vi "read_config_file.vi"(8 "error in (no error)":errorcluster, 11 "Application Directory":path) -> (0 "error out":errorcluster, 1 "gui_strings":string[](array[string]), 2 "devices":T1, 3 "gral_config":T3={"file_ext"="0.0.0.0", "TCP port"=0, "#devices"=0, "log?"=FALSE, "tcp?"=FALSE, "language"="ENG"})   [LabVIEW 2013]
doc: "Reads the configuration file (config.ini)"
uses:
  type_def/general.ctl
  type_def/device_array.ctl
  type_def/device.ctl
  <vilib>/Utility/config.llb/Read Key (I32).vi
  <vilib>/Utility/config.llb/Read Key (Boolean).vi
  <vilib>/Utility/config.llb/Read Key (String).vi
  <vilib>/Utility/config.llb/Read Key (Path).vi
  <vilib>/Utility/config.llb/NI_LVConfig.lvlib
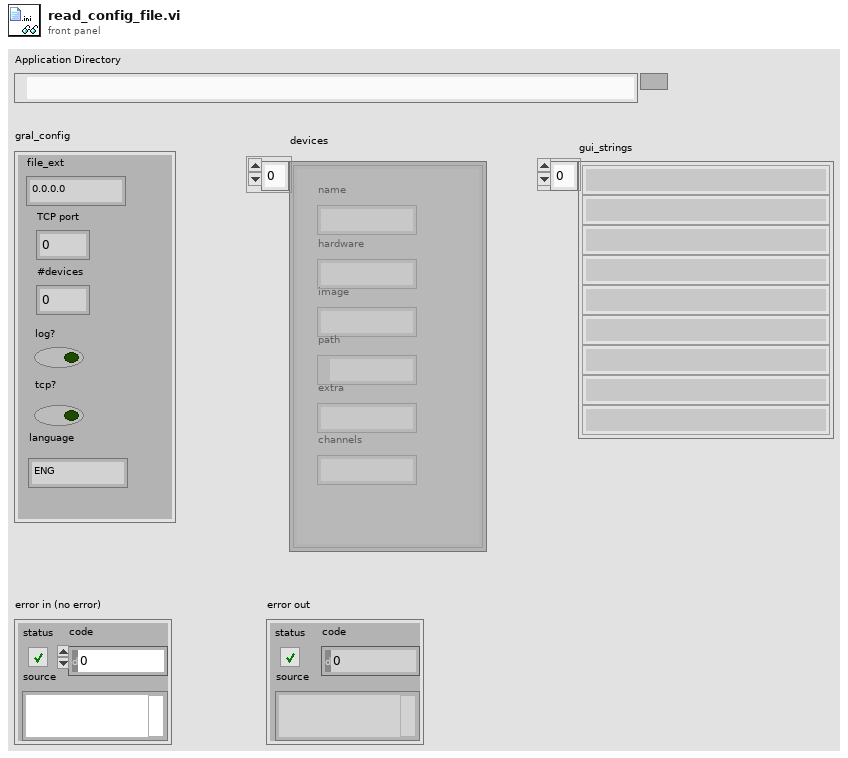
[diagram p1: front panel]
types:
  T1 = typedef "device_array.ctl" = T2[]
  T2 = typedef "device.ctl" = cluster{"name":string, "hardware":string, "image":string, "path":path, "extra":string, "channels":string}
  T3 = typedef "general.ctl" = cluster{"file_ext":string, "TCP port":i32, "#devices":i32, "log?":bool, "tcp?":bool, "language":string}
  T4 = typedef "NI_LVConfig.lvlib/Config Data RefNum.ctl" = refnum<k1>
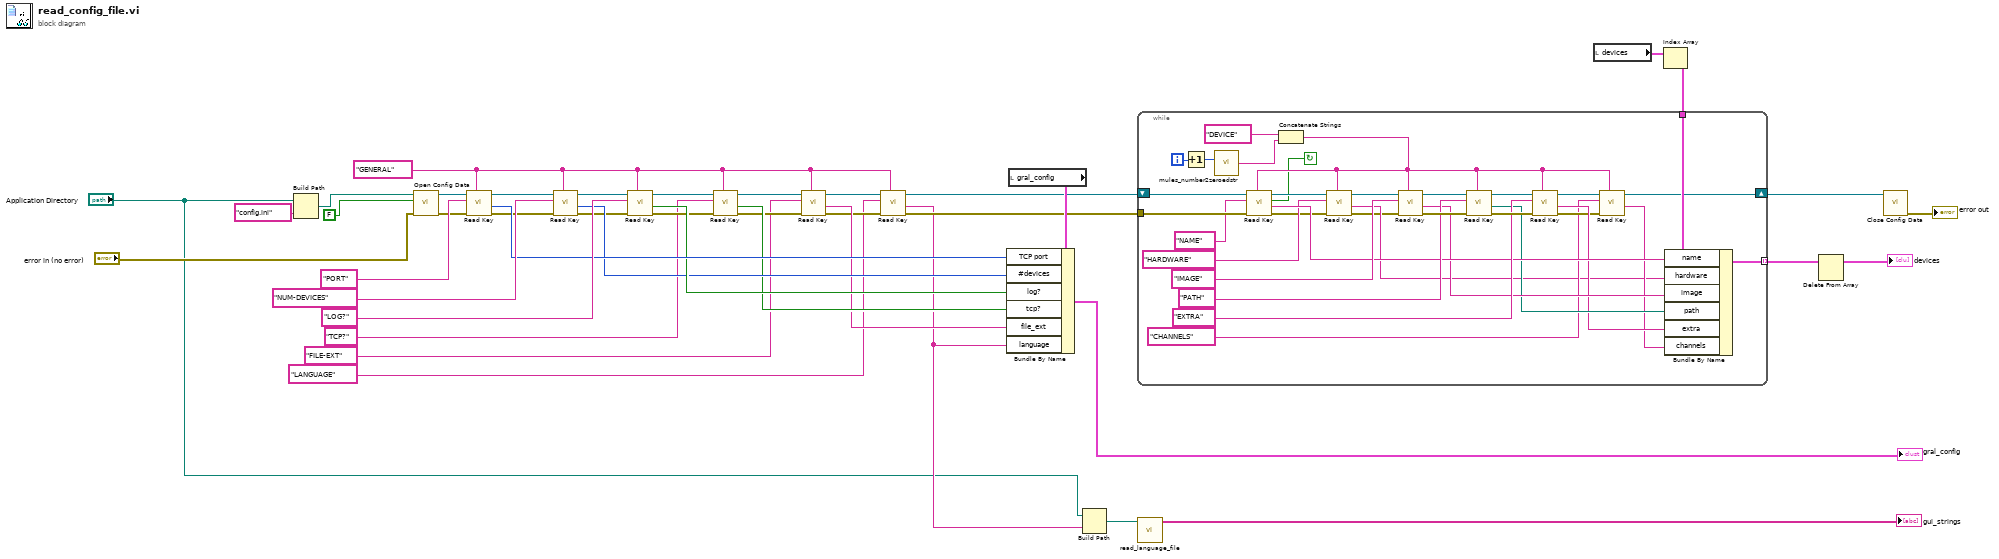
[diagram p0: block diagram]
diagram:
  w13 = "GENERAL" ("section")
  n1 = Build Path(base path="Application Directory", name or relative path="config.ini") -> (appended path=w41:path)
  n2 = call <vilib>:"Open Config Data.vi"("error in (no error)"="error in (no error)", "create file if necessary (T)"=FALSE, "configuration file path"=w41) -> ("error out"=w6:errorcluster, "refnum"=w9:T4)  [unwired: 6 in, 1 out]
  n3 = call-poly <vilib>:"Read Key.vi"("section"=w13, "error in (no error)"=w6, "key"="PORT", "refnum"=w9) -> ("error out"=w7:errorcluster, "value"=w33:i32, "refnum out"=w8:T4)  [unwired: 4 in, 1 out]
  n4 = call-poly <vilib>:"Read Key.vi"("section"=w13, "error in (no error)"=w7, "key"="NUM-DEVICES", "refnum"=w8) -> ("error out"=w27:errorcluster, "value"=w31:i32, "refnum out"=w37:T4)  [unwired: 4 in, 1 out]
  n5 = call-poly <vilib>:"Read Key.vi"("section"=w13, "error in (no error)"=w27, "key"="LOG?", "refnum"=w37) -> ("error out"=w24:errorcluster, "value"=w32:bool, "refnum out"=w25:T4)  [unwired: 4 in, 1 out]
  n6 = call-poly <vilib>:"Read Key.vi"("section"=w13, "error in (no error)"=w24, "key"="TCP?", "refnum"=w25) -> ("error out"=w20:errorcluster, "value"=w22:bool, "refnum out"=w21:T4)  [unwired: 4 in, 1 out]
  n7 = call-poly <vilib>:"Read Key.vi"("section"=w13, "error in (no error)"=w20, "key"="FILE-EXT", "refnum"=w21) -> ("error out"=w17:errorcluster, "value"=w18:string, "refnum out"=w14:T4)  [unwired: 4 in, 1 out]
  n8 = call-poly <vilib>:"Read Key.vi"("section"=w13, "error in (no error)"=w17, "key"="LANGUAGE", "refnum"=w14) -> ("error out"=w16:errorcluster, "value"=w4:string, "refnum out"=w15:T4)  [unwired: 4 in, 1 out]
  n9 = local read "gral_config"() -> (w34:T3)
  n10 = Bundle By Name(cluster=w34, "TCP port"=w33, "#devices"=w31, "log?"=w32, "tcp?"=w22, "file_ext"=w18, "language"=w4) -> (→"gral_config":T3)
  n11 = Build Path(base path="Application Directory", name or relative path=w4) -> (appended path=w5:path)
  n12 = call "read_language_file.vi"("Text File"=w5) -> ("gui_strings"=→"gui_strings":string[])  [unwired: 10 in]
  n13 = local read "devices"() -> (w30:T1)
  n14 = Index Array(array=w30) -> (element=w29:T2)  [unwired: 1 in]
  n15 = while {
    shift-right: [w54] -> w38
    shift-left: w15 -> [w73]
    tunnel: w29 -> [w61]
    tunnel: [w60] -> w11 mode=indexing
    tunnel: w16 -> [w68]
    i -> [w75]
    stop <- w43 continue-if-true
    n16 = Increment(x=w75) -> (x+1=w74:i32)
    n17 = call "mules_number2zeroedstr.vi"("number"=w74) -> ("string"=w62:string)  [unwired: 1 in]
    n18 = Concatenate Strings("DEVICE" ("key"), w62) -> (w48:string)
    n19 = call-poly <vilib>:"Read Key.vi"("section"=w48, "error in (no error)"=w68, "key"="NAME", "refnum"=w73) -> ("error out"=w45:errorcluster, "value"=w59:string, "found?"=w43:bool, "refnum out"=w50:T4)  [unwired: 4 in]
    n20 = call-poly <vilib>:"Read Key.vi"("section"=w48, "error in (no error)"=w45, "key"="HARDWARE", "refnum"=w50) -> ("error out"=w44:errorcluster, "value"=w46:string, "refnum out"=w49:T4)  [unwired: 4 in, 1 out]
    n21 = call-poly <vilib>:"Read Key.vi"("section"=w48, "error in (no error)"=w44, "key"="IMAGE", "refnum"=w49) -> ("error out"=w69:errorcluster, "value"=w58:string, "refnum out"=w72:T4)  [unwired: 4 in, 1 out]
    n22 = call-poly <vilib>:"Read Key.vi"("section"=w48, "error in (no error)"=w69, "key"="PATH", "refnum"=w72) -> ("error out"=w70:errorcluster, "value"=w57:path, "refnum out"=w71:T4)  [unwired: 4 in, 1 out]
    n23 = call-poly <vilib>:"Read Key.vi"("section"=w48, "error in (no error)"=w70, "key"="EXTRA", "refnum"=w71) -> ("error out"=w55:errorcluster, "value"=w56:string, "refnum out"=w53:T4)  [unwired: 4 in, 1 out]
    n24 = call-poly <vilib>:"Read Key.vi"("section"=w48, "error in (no error)"=w55, "key"="CHANNELS", "refnum"=w53) -> ("value"=w51:string, "refnum out"=w54:T4)  [unwired: 4 in, 2 out]
    n25 = Bundle By Name(cluster=w61, "name"=w59, "hardware"=w46, "image"=w58, "path"=w57, "extra"=w56, "channels"=w51) -> (w60:T2)
  }
  n26 = Delete From Array(array=w11) -> (array with subset deleted=→"devices":T2[])  [unwired: 2 in, 1 out]
  n27 = call <vilib>:"Close Config Data.vi"("refnum"=w38) -> ("error out"=→"error out":errorcluster)  [unwired: 9 in, 1 out]
